vi "Latihan 16 (Equation Numerator Denumerator).vi"() -> ()   [LabVIEW 2021]
uses:
  <vilib>/Analysis/polynomials.llb/Add Rational Polynomials (DBL).vi
  <vilib>/addons/Control Design/_Model Construction/Model Creation.llb/Model Creation SubVI/cd_Create Transfer Function Model.vi
  <vilib>/addons/Control Design/_Utility/Model Viewer.llb/Model Viewer SubVI/cd_Draw Transfer Function Equation (TF).vi
  <vilib>/Analysis/NI_AALPro.lvlib
  <vilib>/addons/Control Design/_Model Construction/NI_LinSys_Model Creation.lvlib
  <vilib>/addons/Control Design/_Utility/NI_CD_Model Viewer.lvlib
panel:
  in  "Denominator 2":dbl[](array[numeric]) format="%#.2g"
  in  "Numerator 2":dbl[](array[numeric]) format="%#.2g"
  in  "Denominator 1":dbl[](array[numeric]) format="%#.2g"
  in  "Numerator 1":dbl[](array[numeric]) format="%#.2g"
  out "Equation":picture
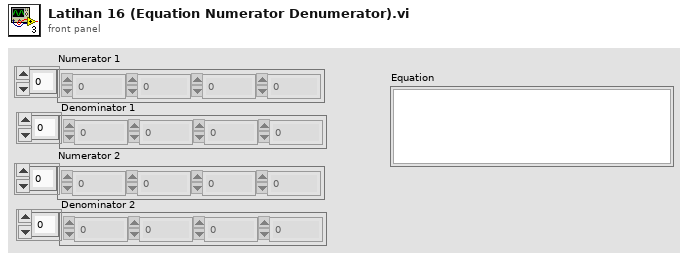
[diagram p1: front panel]
types:
  T1 = typedef "NI_LinSys_Model Typedefs.lvlib/CD Transfer Function Model (MIMO).ctl" = cluster{"properties":T2, "transfer function(s)":T3[][]}
  T2 = typedef "NI_LinSys_Model Typedefs.lvlib/CD General Elements.ctl" = cluster{"Model name":string, "Input names":string[], "Output names":string[], "Input Delays":dbl[], "Output Delays":dbl[], "Sampling Time":dbl, "Notes":string}
  T3 = typedef "NI_LinSys_Model Typedefs.lvlib/CD Transfer Function Model (SISO).ctl" = cluster{"Numerator":dbl[], "Denominator":dbl[], "delay":dbl}
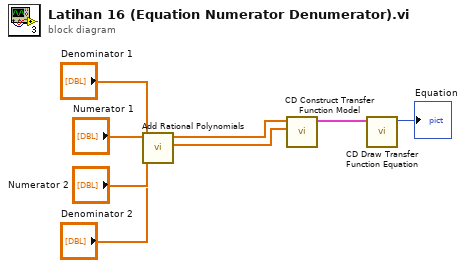
[diagram p0: block diagram]
diagram:
  n1 = call-poly <vilib>:"Add Rational Polynomials.vi"("Denominator 2"="Denominator 2", "Numerator 2"="Numerator 2", "Denominator 1"="Denominator 1", "Numerator 1"="Numerator 1") -> ("Denominator Out"=w7:dbl[], "Numerator Out"=w8:dbl[])  [unwired: 5 in, 1 out]
  n2 = call-poly <vilib>:"CD Construct Transfer Function Model.vi"("Denominator"=w7, "Numerator"=w8) -> ("Transfer Function Model"=w6:T1)  [unwired: 8 in, 1 out]
  n3 = call-poly <vilib>:"CD Draw Transfer Function Equation.vi"("Transfer Function Model"=w6) -> ("Equation"=→"Equation":picture)  [unwired: 8 in, 2 out]
